vi "Register Events to Controller.vi"(8 "error in (no error)":errorcluster, 11 "Example View in":refnum<class "Example View.lvclass">) -> (0 "error out":errorcluster, 3 "Example View out":refnum<class "Example View.lvclass">)   [LabVIEW 2023, in "Example MVC Actors.lvlib" / "Example View.lvlib" / "Example View.lvclass"]
doc: "This dinamic dispatch methods has to be overriddent by the child sink classes to register events to the source"
uses:
  Example View.lvclass
  C:/Projects/Shared Libraries/Event Actors/View/View.lvclass
  Example Events/Double Array Event.lvclass
  C:/Projects/Shared Libraries/Event Actors/Event/Event.lvclass
  Example Events/Timestamp Event.lvclass
  Example View Messages/Update Array Event Msg/Update Array Event Msg.lvclass
  C:/Projects/Shared Libraries/Event Actors/Event Handlers/Abstract Event Message for View/Abstract Event Message for View.lvclass
  Example View Messages/Update Time Event Msg/Update Time Event Msg.lvclass
  Example View Messages/Update Boolean Event Msg/Update Boolean Event Msg.lvclass
  Example Events/Boolean Event.lvclass
  Example Events/Inited At Event.lvclass
  Example View Messages/Update Inited At Event Msg/Update Inited At Event Msg.lvclass
  Event/Event.lvclass/Event.ctl
  Event/Event.lvclass
  View/View.lvclass
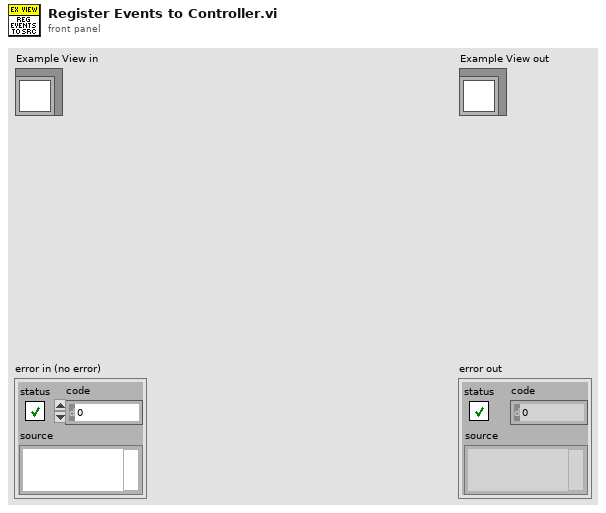
[diagram p1: front panel]
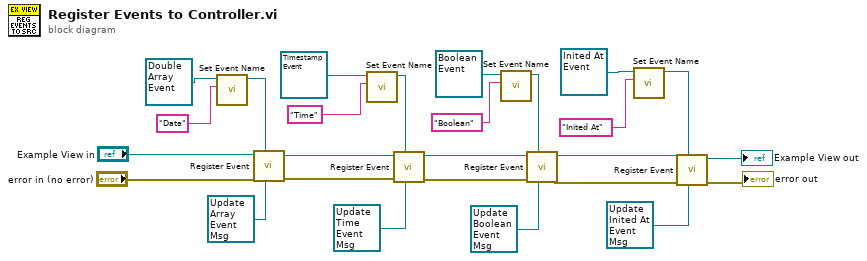
[diagram p0: block diagram]
diagram:
  n1 = call "Set Event Name.vi"("Name (Generic)"="Data", "Event In"=refnum<class "Double Array Event.lvclass"> refnum ("Double Array Event.lvclass")) -> ("Event Out"=w22:refnum<class "Double Array Event.lvclass">)  [unwired: 9 in]
  n2 = call "Register Event.vi"("Event Handler"=refnum<class "Update Array Event Msg.lvclass"> refnum ("Update Array Msg.lvclass"), "Event"=w22, "error in (no error)"="error in (no error)", "View Actor in"="Example View in") -> ("error out"=w17:errorcluster, "View Actor out"=w18:refnum<class "Example View.lvclass">)  [unwired: 6 in]
  n3 = call "Set Event Name.vi"("Name (Generic)"="Time", "Event In"=refnum<class "Timestamp Event.lvclass"> refnum ("Timestamp Event.lvclass")) -> ("Event Out"=w19:refnum<class "Timestamp Event.lvclass">)  [unwired: 9 in]
  n4 = call "Register Event.vi"("Event Handler"=refnum<class "Update Time Event Msg.lvclass"> refnum ("Update Time Msg.lvclass"), "Event"=w19, "error in (no error)"=w17, "View Actor in"=w18) -> ("error out"=w10:errorcluster, "View Actor out"=w11:refnum<class "Example View.lvclass">)  [unwired: 6 in]
  n5 = call "Set Event Name.vi"("Name (Generic)"="Boolean", "Event In"=refnum<class "Boolean Event.lvclass"> refnum ("Example Source.lvlib:Boolean Event.lvclass")) -> ("Event Out"=w12:refnum<class "Boolean Event.lvclass">)  [unwired: 9 in]
  n6 = call "Register Event.vi"("Event Handler"=refnum<class "Update Boolean Event Msg.lvclass"> refnum ("Update Time Msg.lvclass"), "Event"=w12, "error in (no error)"=w10, "View Actor in"=w11) -> ("error out"=w4:errorcluster, "View Actor out"=w5:refnum<class "Example View.lvclass">)  [unwired: 6 in]
  n7 = call "Set Event Name.vi"("Name (Generic)"="Inited At", "Event In"=refnum<class "Inited At Event.lvclass"> refnum ("Inited At Event.lvclass")) -> ("Event Out"=w6:refnum<class "Inited At Event.lvclass">)  [unwired: 9 in]
  n8 = call "Register Event.vi"("Event Handler"=refnum<class "Update Inited At Event Msg.lvclass"> refnum ("Example View Actor.lvlib:Update Updated At Event Msg.lvclass"), "Event"=w6, "error in (no error)"=w4, "View Actor in"=w5) -> ("error out"=→"error out":errorcluster, "View Actor out"=→"Example View out":refnum<class "Example View.lvclass">)  [unwired: 6 in]
